vi "GoalieErrorHistogram.vi"(11 "IA state":T1={"our_robots"=[], "enemy_robots"=[], "balls"=[], "geometry"={"line_width"=0, "field_length"=0, "field_width"=0, "boundary_width"=0, "referee_width"=0, "goal_width"=0, "goal_depth"=0, "goal_wall_width"=0, "center_circle_radius"=0, "defense_radius"=0, "defense_stretch"=0, "free_kick_from_defense_dist"=0, "penalty_spot_from_field_line_dist"=0, "penalty_line_from_spot_dist"=0}, "IA Judge"={"stage"="", "command"="", "our_goalie_id"=0.0, "enemy_goalie_id"=0.0, "command enum"=enum."Halt", "Time"=enum."Azul"}, "Received Timestamp"=timestamp(0 s since 1904-01-01), "Events"={"Touch"=FALSE, "Ball out"=FALSE, "id touch"=0.0, "Ball out of \nVision"=FALSE, "Ball inside \nGoalie area"=FALSE, "Robot not responding"=FALSE, "Robots responding status"=[1.0, 1.0, 1.0, 1.0, 1.0, 1.0], "Enemy Ball \nPossession"=FALSE, "Pass State"=FALSE, "id end of pass"=0.0, "Kick"=FALSE, "Id ini Possession"=0.0, "Ball Possesion"=FALSE, "Id Possesion"=0.0}}) -> (3 "Goalie Error Histogram":cluster{dbl[], dbl[]}(graph))   [LabVIEW 2017]
uses:
  Core/AI Input.ctl
  Core/AI Robot.ctl
  Intel/Functions Enum.ctl
  Intel/AttackerStates.ctl
  Core/AI Ball.ctl
  Core/Field Size.ctl
  Core/AI Judge.ctl
  Intel/Command Enum.ctl
  Util/Events/Events.ctl
panel:
  out "Goleiro ultimo com a bola":bool=TRUE
  in  "Divisões do gol":i32=20
  out "Array":dbl[](array[numeric])
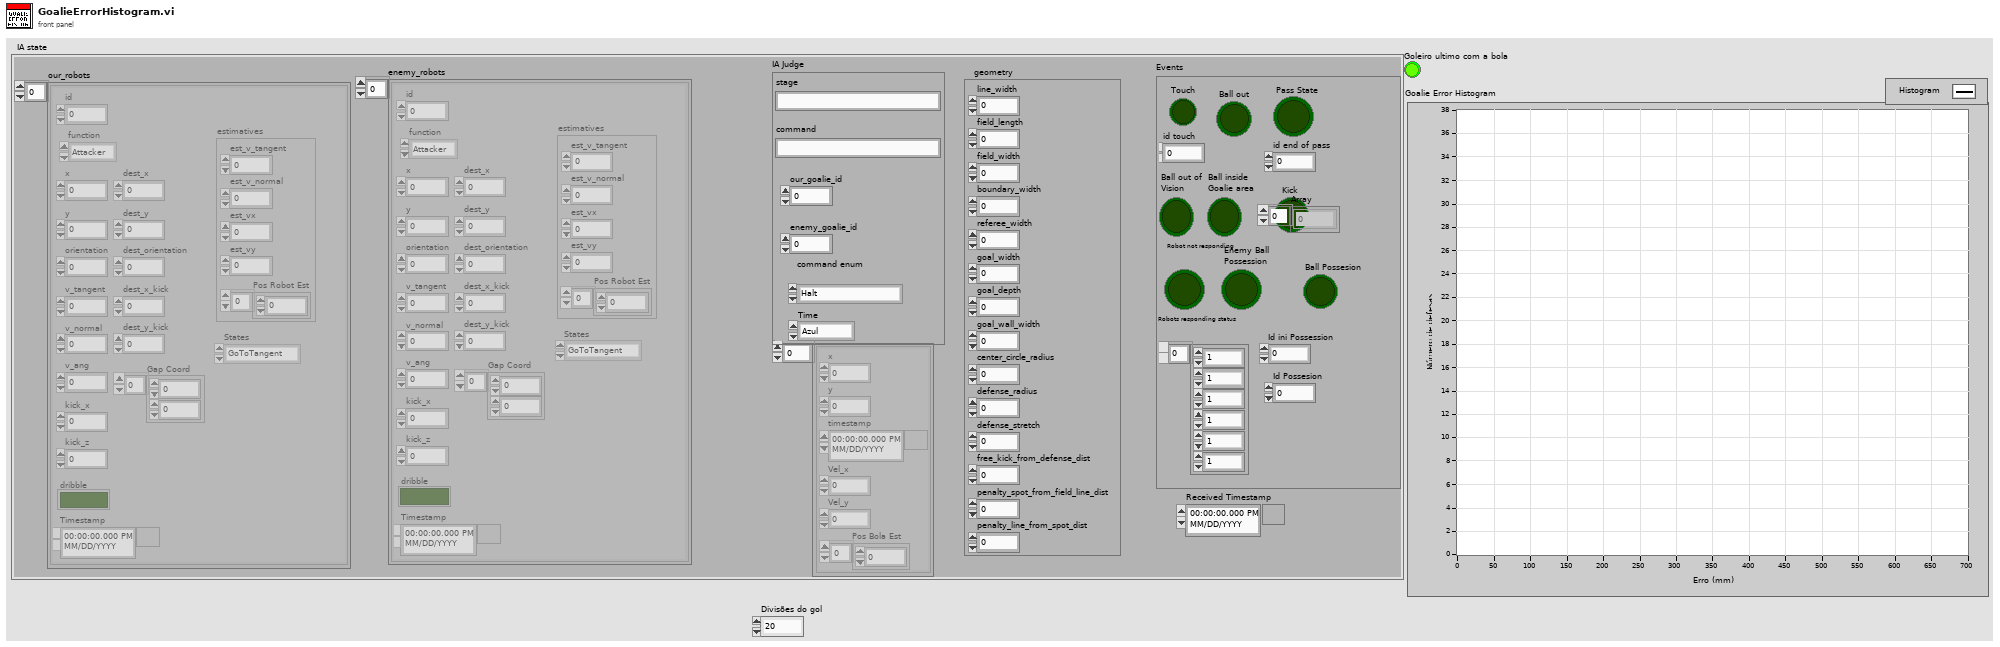
[diagram p1: front panel]
types:
  T1 = typedef "AI Input.ctl" = cluster{"our_robots":T2[], "enemy_robots":T2[], "balls":T5[], "geometry":T6, "IA Judge":T7, "Received Timestamp":timestamp, "Events":T9}
  T2 = typedef "AI Robot.ctl" = cluster{"id":u32, "function":T3, "x":dbl, "y":dbl, "orientation":dbl, "v_tangent":dbl, "v_normal":dbl, "v_ang":dbl, "kick_x":dbl, "kick_z":dbl, "dribble":bool, "Timestamp":timestamp, "dest_x":dbl, "dest_y":dbl, "dest_orientation":dbl, "estimatives":cluster{"est_v_tangent":dbl, "est_v_normal":dbl, "est_vx":dbl, "est_vy":dbl, "Pos Robot Est":dbl[]}, "dest_x_kick":dbl, "dest_y_kick":dbl, "Gap Coord":dbl[], "States":T4}
  T3 = typedef "Functions Enum.ctl" = enum16{"Attacker", "Goalie", "Defender", "Striker", "Goto 0", "Dummy", "Kicker", "ZigZag"}
  T4 = typedef "AttackerStates.ctl" = enum16{"Pass", "GoToTangent", "BallGetting", "GoToKick", ""}
  T5 = typedef "AI Ball.ctl" = cluster{"x":dbl, "y":dbl, "timestamp":timestamp, "Vel_x":dbl, "Vel_y":dbl, "Pos Bola Est":dbl[]}
  T6 = typedef "Field Size.ctl" = cluster{"line_width":u32, "field_length":u32, "field_width":u32, "boundary_width":u32, "referee_width":u32, "goal_width":u32, "goal_depth":u32, "goal_wall_width":u32, "center_circle_radius":u32, "defense_radius":u32, "defense_stretch":u32, "free_kick_from_defense_dist":u32, "penalty_spot_from_field_line_dist":u32, "penalty_line_from_spot_dist":u32}
  T7 = typedef "AI Judge.ctl" = cluster{"stage":string, "command":string, "our_goalie_id":dbl, "enemy_goalie_id":dbl, "command enum":T8, "Time":enum16{"Azul", "Amarelo"}}
  T8 = typedef "Command Enum.ctl" = enum16{"Halt", "Stop", "Force Start", "PKA Normal Start", "Prepare Kickoff Ally", "PKE Normal Start", "Prepare Kickoff Enemy", "Prepare Penalty Ally", "PPA Normal Start", "Prepare Penalty Enemy", "PPE Normal Start", "Direct Free Enemy", "Direct Free Ally", "Indirect Free Enemy", "Indirect Free Ally", "Timeout Enemy", "Timeout Ally", "Goal Enemy", "Goal Ally", "Ball Placement Enemy", "Ball Placement Ally", "Normal Half Time", "Extra Time Break", "Extra Half Time", "None", "Post Game"}
  T9 = typedef "Events.ctl" = cluster{"Touch":bool, "Ball out":bool, "id touch":dbl, "Ball out of \nVision":bool, "Ball inside \nGoalie area":bool, "Robot not responding":bool, "Robots responding status":dbl[], "Enemy Ball \nPossession":bool, "Pass State":bool, "id end of pass":dbl, "Kick":bool, "Id ini Possession":dbl, "Ball Possesion":bool, "Id Possesion":dbl}
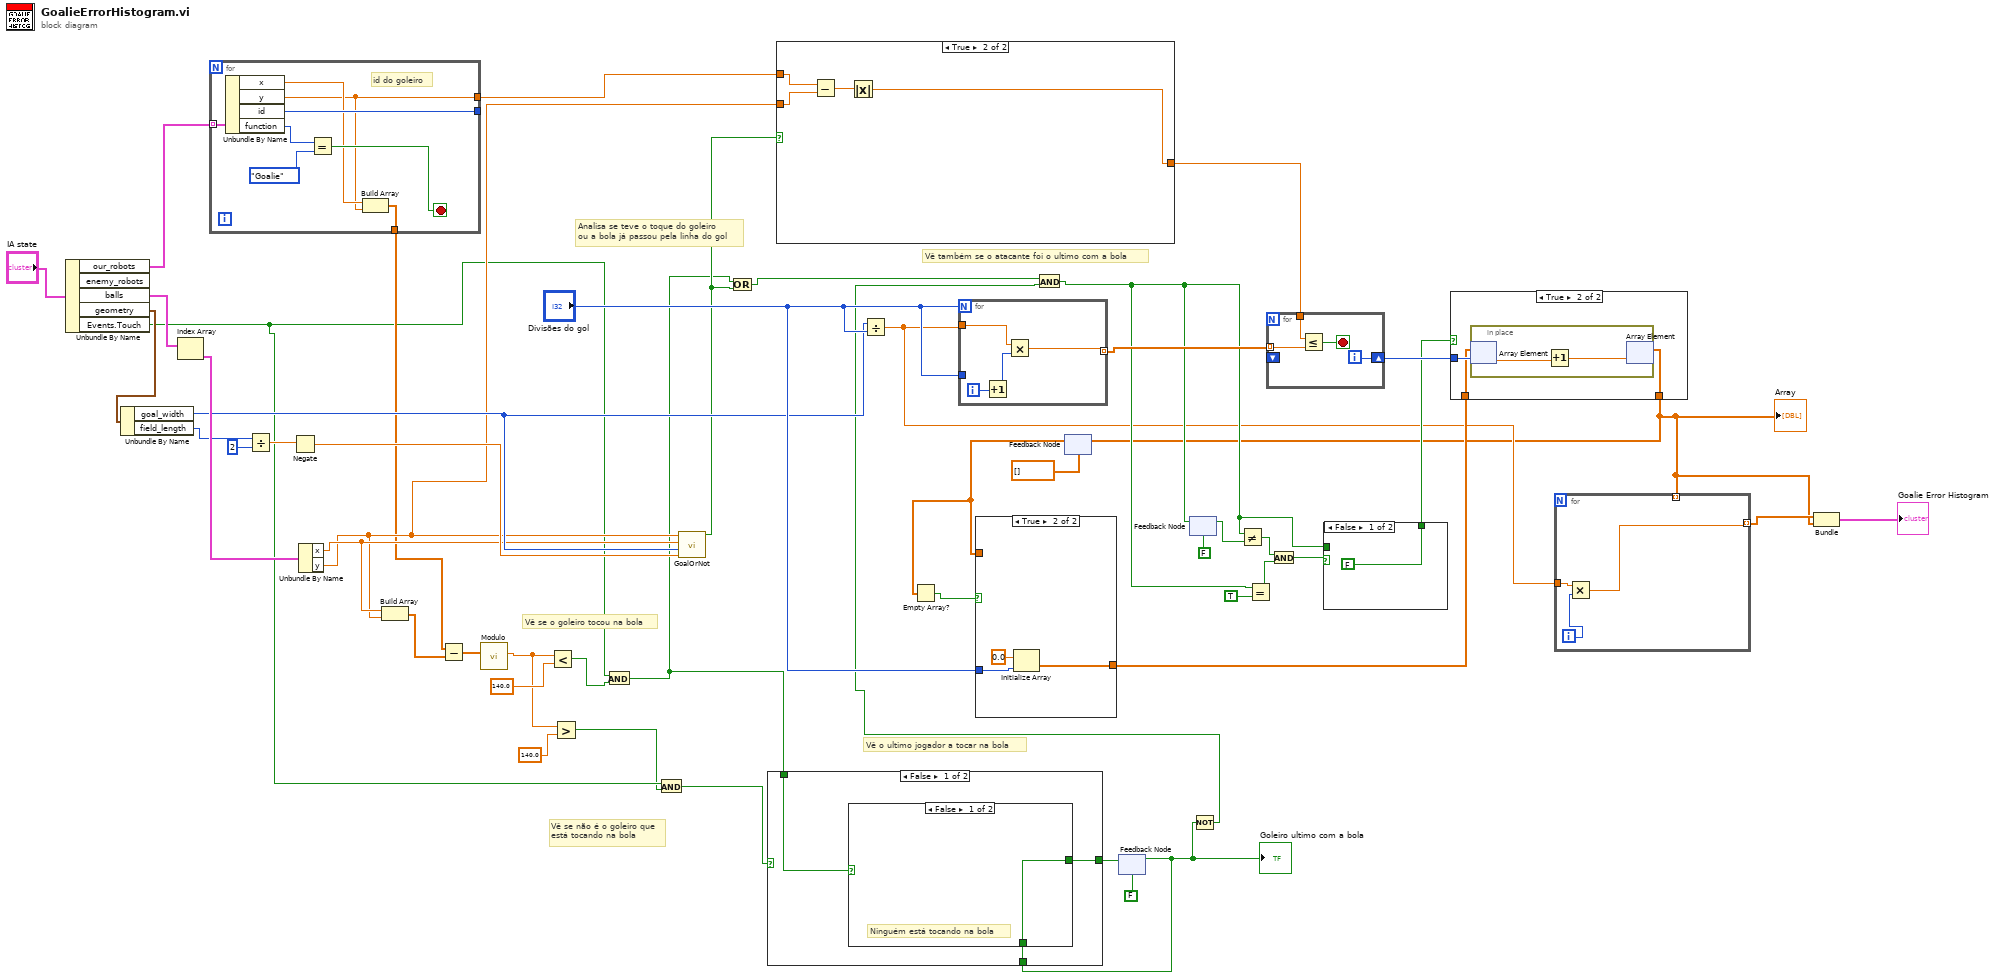
[diagram p0: block diagram]
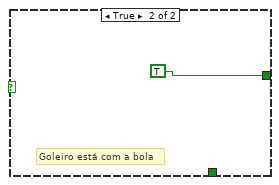
[diagram p3: hidden frame]
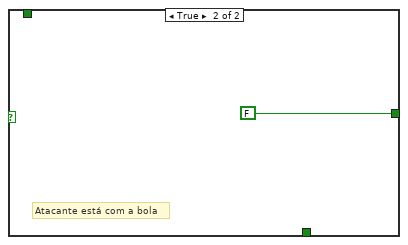
[diagram p4: hidden frame]
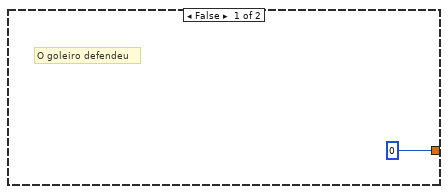
[diagram p6: hidden frame]
diagram:
  # "Vê também se o atacante foi o ultimo com a bola"
  # "Vê o ultimo jogador a tocar na bola"
  # "Vê se não é o goleiro que\nestá tocando na bola"
  # "Vê se o goleiro tocou na bola"
  # "Analisa se teve o toque do goleiro\nou a bola já passou pela linha do gol"
  n1 = Unbundle By Name("IA state") -> ("our_robots"=w49:T2[], "balls"=w48:T5[], "geometry"=w46:T6, "Events.Touch"=w23:bool)  [unwired: 1 out]
  n2 = Unbundle By Name(w46) -> ("goal_width"=w36:u32, "field_length"=w45:u32)
  n3 = Index Array(array=w48) -> (element=w47:T5)  [unwired: 1 in]
  n4 = for {
    tunnel: w49 -> [w58] mode=indexing
    tunnel: [w54] -> _
    tunnel: [w52] -> w34
    tunnel: [w51] -> w28
    stop <- w55 stop-if-true
    # "id do goleiro"
    n5 = Unbundle By Name(w58) -> ("x"=w53:dbl, "y"=w52:dbl, "id"=w54:u32, "function"=w57:T3)
    n6 = Equal?(x=w57, y=Functions_Enum."Goalie") -> (x = y?=w55:bool)
    n7 = Build Array(w53, w52) -> (w51:dbl[])
  }
  n8 = Divide(x=w45, y=u32 2) -> (x/y=w33:dbl)
  n9 = Negate(x=w33) -> (-x=w32:dbl)
  n10 = Unbundle By Name(w47) -> ("x"=w30:dbl, "y"=w29:dbl)
  n11 = Build Array(w30, w29) -> (w27:dbl[])
  n12 = Subtract(x=w28, y=w27) -> (x-y=w26:dbl[])
  n13 = call "Modulo.vi"("2D vector"=w26) -> ("Modulo"=w21:dbl)  [unwired: 10 in]
  n14 = Less?(x=w21, y=140.0) -> (x < y?=w24:bool)
  n15 = Greater?(x=w21, y=140.0) -> (0:w20:bool)
  n16 = And(x=w23, y=w24) -> (x .and. y?=w18:bool)
  n17 = And(x=w23, y=w20) -> (x .and. y?=w19:bool)
  n18 = call "GoalOrNot.vi"("goal x"=w32, "goal width"=w36, "ball x"=w30, "ball y"=w29) -> ("Goal or Not"=w31:bool)  [unwired: 7 in]
  n19 = Or(x=w18, y=w31) -> (x .or. y?=w6:bool)
  n20 = case shown="True" w31 {
    tunnel: [0 w60] -> w35
    tunnel: w34 -> [_ w63]
    tunnel: w29 -> [_ w62]
    frame False {
      # "O goleiro defendeu"
    }
    frame True {
      n21 = Subtract(x=w63, y=w62) -> (x-y=w61:dbl)
      n22 = Absolute Value(x=w61) -> (abs(x)=w60:dbl)
    }
  }
  n23 = Divide(x=w36, y="Divisões do gol") -> (x/y=w4:dbl)
  n24 = for {
    N: "Divisões do gol" -> [_]
    tunnel: w4 -> [w67]
    tunnel: "Divisões do gol" -> [_]
    tunnel: [w66] -> w43 mode=indexing
    i -> [w65]
    n25 = Increment(x=w65) -> (x+1=w64:i32)
    n26 = Multiply(x=w67, y=w64) -> (x*y=w66:dbl)
  }
  n27 = feedback #1(dbl[] []) -> (w40:dbl[])
  n28 = Empty Array?(array=w40) -> (empty?=w39:bool)
  n29 = case shown="True" w39 {
    tunnel: w40 -> [w68 _]
    tunnel: [w68 w70] -> w38
    tunnel: "Divisões do gol" -> [_ w69]
    frame False {
    }
    frame True {
      n30 = Initialize Array(0.0 ("element"), w69) -> (w70:dbl[])
    }
  }
  n31 = feedback #2(FALSE) -> (w8:bool)
  "Goleiro ultimo com a bola" <- w8
  n32 = case shown="False" w19 {
    tunnel: w18 -> [w74 _]
    tunnel: [w73 FALSE] -> w17
    tunnel: w8 -> [w72 _]
    frame False {
      n33 = case shown="False" w74 {
        tunnel: [w75 TRUE] -> w73
        tunnel: w72 -> [w75 _]
        frame False {
          # "Ninguém está tocando na bola"
        }
        frame True {
          # "Goleiro está com a bola"
        }
      }
    }
    frame True {
      # "Atacante está com a bola"
    }
  }
  n34 = feedback-in #2(w17) -> ()
  n35 = feedback #3(FALSE) -> (w14:bool)
  n36 = Not(x=w8) -> (.not. x?=w7:bool)
  n37 = And(x=w6, y=w7) -> (x .and. y?=w5:bool)
  n38 = feedback-in #3(w5) -> ()
  n39 = Not Equal?(x=w5, y=w14) -> (x != y?=w13:bool)
  n40 = Equal?(x=w5, y=TRUE) -> (x = y?=w11:bool)
  n41 = for {
    shift-right: [w80] -> w42
    shift-left: _ -> [_]
    tunnel: w43 -> [w79] mode=indexing
    tunnel: w35 -> [w78]
    i -> [w80]
    stop <- w81 stop-if-true
    n42 = Less Or Equal?(x=w78, y=w79) -> (x <= y?=w81:bool)
  }
  n43 = And(x=w13, y=w11) -> (x .and. y?=w10:bool)
  n44 = case shown="False" w10 {
    tunnel: [FALSE w83] -> w9
    tunnel: w5 -> [_ w83]
    frame False {
    }
    frame True {
    }
  }
  n45 = case shown="True" w9 {
    tunnel: w42 -> [_ w87]
    tunnel: w38 -> [w84 w86]
    tunnel: [w84 w85] -> w2
    frame False {
    }
    frame True {
      n46 = in-place {
        n47 = in-place-array #4(w86, w87) -> (w89:dbl)
        n48 = Increment(x=w89) -> (x+1=w88:dbl)
        n49 = in-place-array #4(w88) -> (w85:dbl[])  [unwired: 1 out]
      }
    }
  }
  "Array" <- w2
  n50 = feedback-in #1(w2) -> ()
  n51 = for {
    tunnel: [w91] -> w3 mode=indexing
    tunnel: w4 -> [w90]
    tunnel: w2 -> [_] mode=indexing
    i -> [w92]
    n52 = Multiply(x=w90, y=w92) -> (x*y=w91:dbl)
  }
  n53 = Bundle(w3, w2) -> (→"Goalie Error Histogram":cluster{dbl[], dbl[]})  [unwired: 1 in]
